vi "Close.vi"(8 "error in (no error)":errorcluster, 11 "TCP Connection in":refnum<class "TCP Connection.lvclass">) -> (0 "error out":errorcluster)   [LabVIEW 2017, in "TCP Interface.lvlib" / "TCP Connection.lvclass"]
uses:
  <vilib>/gpm_packages/@cs/Network-sink/Source/TCP Interface/TCP Connection/TCP Connection.lvclass
  <vilib>/gpm_packages/@cs/Network-sink/Source/TCP Interface/TCP Connection/TCP Connection.lvclass/TCP Connection.ctl
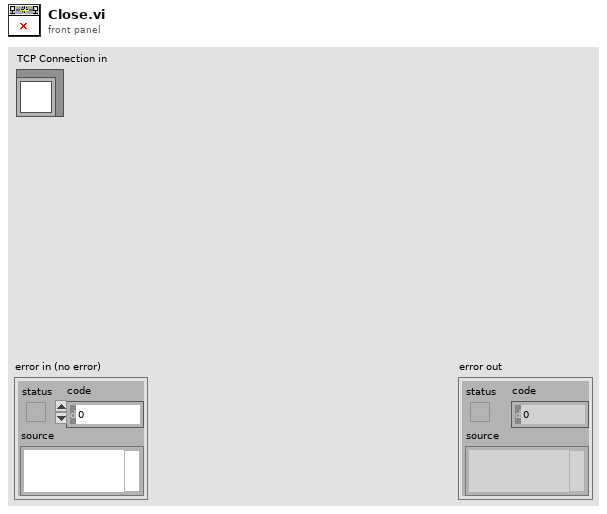
[diagram p1: front panel]
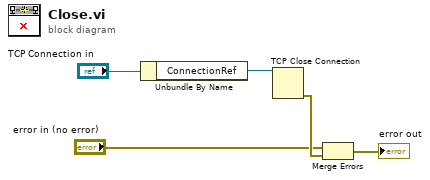
[diagram p0: block diagram]
diagram:
  n1 = Unbundle By Name("TCP Connection in") -> ("ConnectionRef"=w4:refnum<k5>)
  n2 = TCP Close Connection(connection ID=w4) -> (error out=w3:errorcluster)  [unwired: 2 in, 1 out]
  n3 = Merge Errors("error in (no error)", w3) -> (→"error out":errorcluster)
